vi "Configure List Data(Only 7723).vi"(4 "Range":bool, 6 "End State":bool, 7 "Repeat":u32=1 min=1 max=50000 step=1, 8 "error in":errorcluster, 9 "Jump To":u32=1 min=1 max=50 step=1, 10 "Record Num":u32=1 min=1 max=50 step=1, 11 "VISA resource name":refnum<visa-resource-name>) -> (0 "error out":errorcluster, 3 "VISA resource name out":refnum<visa-resource-name>)   [LabVIEW 2015, in "IT-M7700.lvlib"]
doc: "This command is used to set the configuration parameters for each set of lists.The configuration parameter format is: \"List total steps,Jump,Repeat,End State, preserve parameters\".The detailed parameters are described below.\n<b>Record Num</b>\nSet the total number of steps in the current List\n1~50\n<b>Jump To</b>\nSet the number of steps from which the current List should be executed.\n1~50\n<b>Repeat</b>\nSet the number of repeat executions of the current List\n1~50000.\n<b>End State</b>\nSet the output state of the instrument after the execution of the current List\n0 :OFF\n1: ON\n<b>Range</b>\n0: Low range\n1: High range"
uses:
  <instrlib>/IT-M7700/IT-M7700.lvlib
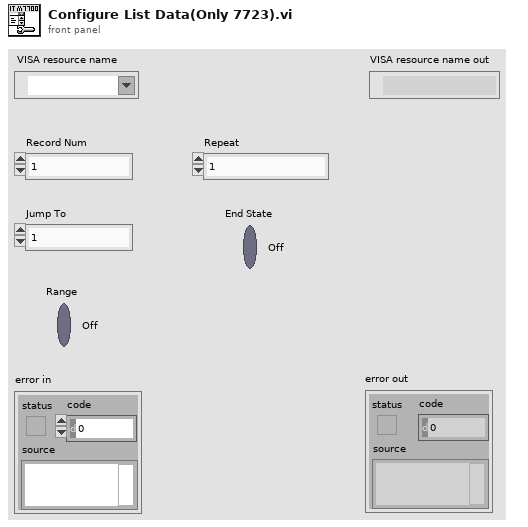
[diagram p1: front panel]
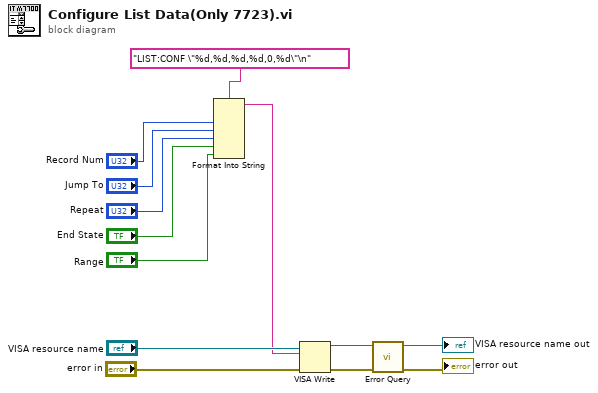
[diagram p0: block diagram]
diagram:
  n1 = Format Into String(format string="LIST:CONF \"%d,%d,%d,%d,0,%d\"\n", "Record Num", "Jump To", "Repeat", "End State", "Range") -> (resulting string=w10:string)  [unwired: 2 in, 1 out]
  n2 = VISA Write(VISA resource name="VISA resource name", write buffer=w10, error in (no error)="error in") -> (VISA resource name out=w9:refnum<visa-resource-name>, error out=w8:errorcluster)  [unwired: 1 out]
  n3 = call <instrlib>:"Error Query.vi"("error in"=w8, "VISA resource name"=w9) -> ("error out"=→"error out":errorcluster, "VISA resource name out"=→"VISA resource name out":refnum<visa-resource-name>)  [unwired: 6 in, 2 out]
